vi "Clear Connections.vi"(8 "error in (no error)":errorcluster, 11 "RT Data Cluster in":T1={"Timekeeper hdl"="", "clkDisc session"=variant, "Compiled Data"={"SyncMod?"=FALSE, "SyncMod"="", "ConnectionSettings"={"Mode"=enum."Generate sample clock", "pxitrig"=FALSE, "pfi0"=FALSE, "pfi1"=FALSE, "pfi2"=FALSE, "External Pin"=enum."PFI0", "Routes"=[]}, "TimeKeeper"="", "ScanOffset(%)"=0.0, "StartDelay(s)"=0, "Time Ref Settings"={"Time Reference"=enum."GPS", "Priority 1"=0, "Priority 2"=0, "IRIG type"=enum."IRIGB AM", "Terminal"="", "PPSSetTime"=FALSE, "Start Time"=timestamp(0 s since 1904-01-01)}, "FIFO Locations"={"BoardTime"=[], "Status"=[]}}, "OutputsData"=[], "OutputsFIFO"=refnum, "Scan Period"=0, "Timekeeper type"=enum."6683", "SyncMod type"=enum."6683", "SyncMod hdl"="", "Custom Device Name"=""} {"Compiled Data"."Time Ref Settings"."Priority 2" min=0 max=255; "Compiled Data"."Time Ref Settings"."Priority 1" min=0 max=255}) -> (0 "error out":errorcluster, 3 "RT Data Cluster out":T1={"Timekeeper hdl"="", "clkDisc session"=variant, "Compiled Data"={"SyncMod?"=FALSE, "SyncMod"="", "ConnectionSettings"={"Mode"=enum."Generate sample clock", "pxitrig"=FALSE, "pfi0"=FALSE, "pfi1"=FALSE, "pfi2"=FALSE, "External Pin"=enum."PFI0", "Routes"=[]}, "TimeKeeper"="", "ScanOffset(%)"=0.0, "StartDelay(s)"=0, "Time Ref Settings"={"Time Reference"=enum."GPS", "Priority 1"=0, "Priority 2"=0, "IRIG type"=enum."IRIGB AM", "Terminal"="", "PPSSetTime"=FALSE, "Start Time"=timestamp(0 s since 1904-01-01)}, "FIFO Locations"={"BoardTime"=[], "Status"=[]}}, "OutputsData"=[], "OutputsFIFO"=refnum, "Scan Period"=0, "Timekeeper type"=enum."6683", "SyncMod type"=enum."6683", "SyncMod hdl"="", "Custom Device Name"=""} {"Compiled Data"."Time Ref Settings"."Priority 2" min=0 max=255; "Compiled Data"."Time Ref Settings"."Priority 1" min=0 max=255})   [LabVIEW 2020, in "NI Synchronization Engine.lvlib"]
uses:
  NI Synchronization Engine.lvlib
  Timekeeper Route Pin.ctl
  <instrlib>/niSync/niSync.llb/niSync Initialize (Default).vi
  niveristand-synchronization-custom-device-2024/Source/Engine/mdevClkDisc.llb/_clkDisc_session.ctl
  Shared/Route.ctl
  Shared/NI Synchronization Shared.lvlib
  Shared/Routes.ctl
  Shared/External Pin.ctl
  Shared/Mode.ctl
  Shared/Connection Settings.ctl
  Shared/IRIG Type.ctl
  Shared/Time Ref Settings.ctl
  Shared/Compiled Data.ctl
  RT Data Cluster.ctl
  Shared/Time Reference.ctl
  timekeeper type.ctl
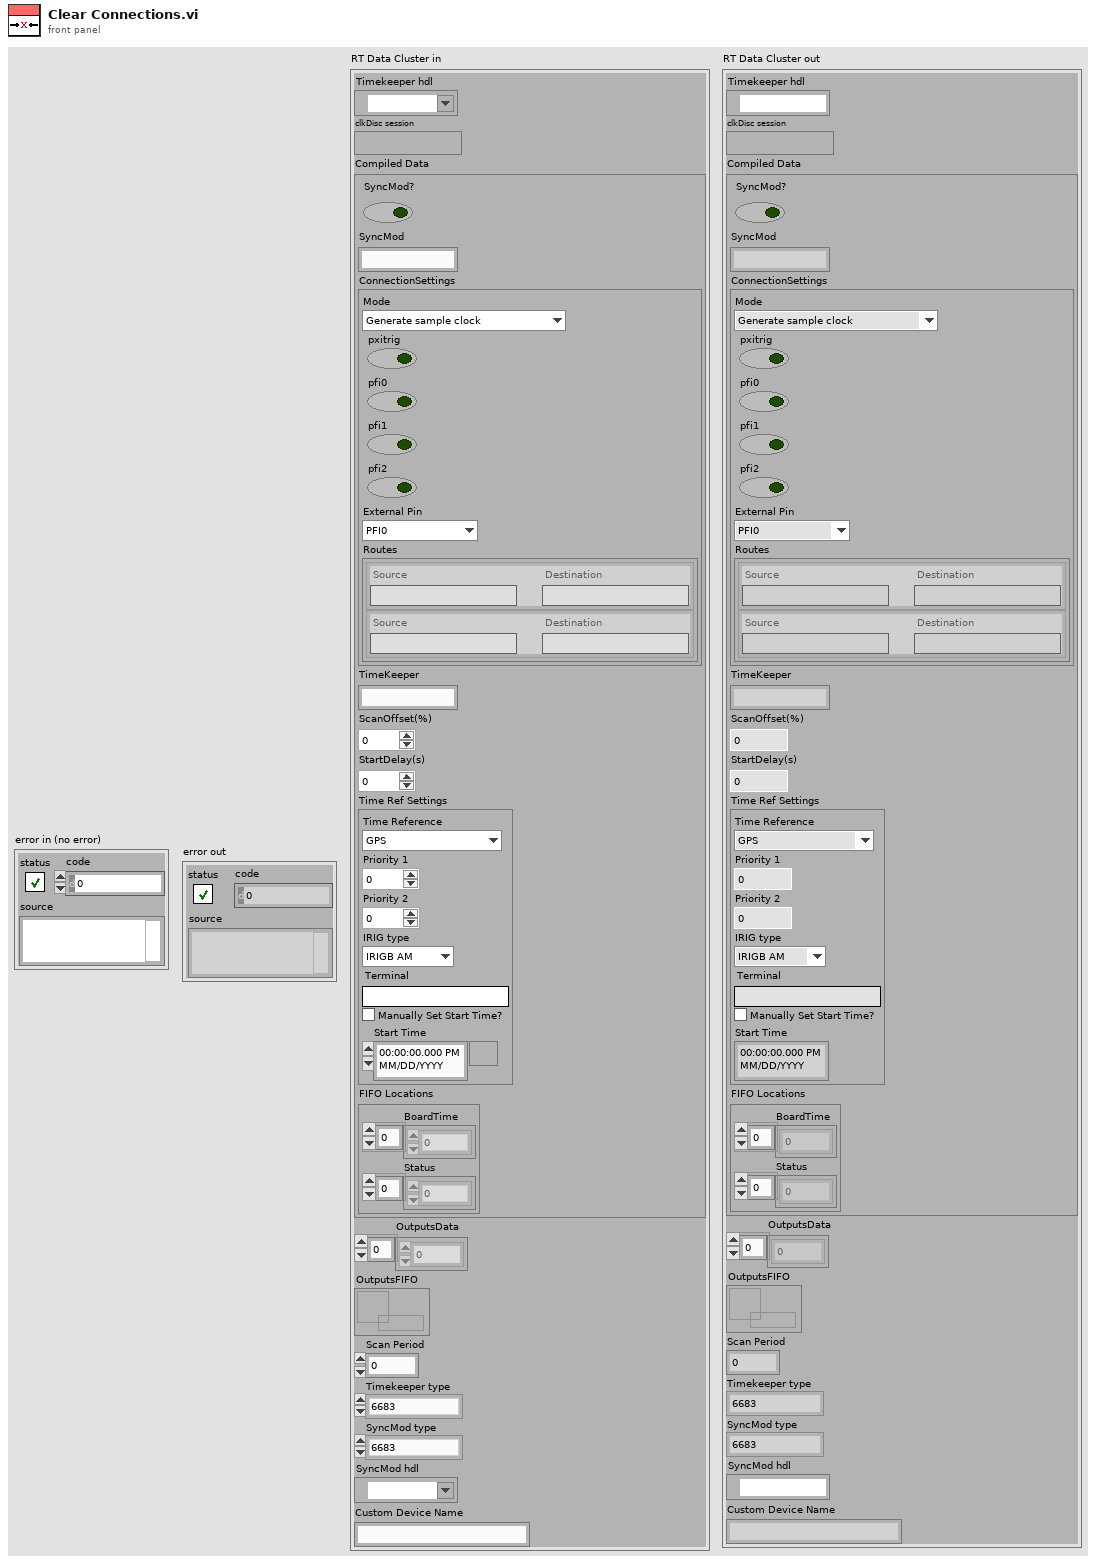
[diagram p1: front panel]
types:
  T1 = typedef "NI Synchronization Engine.lvlib/RT Data Cluster.ctl" = cluster{"Timekeeper hdl":refnum<k15>, "clkDisc session":T2, "Compiled Data":T3, "OutputsData":dbl[], "OutputsFIFO":refnum<k33>, "Scan Period":u32, "Timekeeper type":T12, "SyncMod type":T12, "SyncMod hdl":refnum<k15>, "Custom Device Name":string}
  T2 = typedef "_clkDisc_session.ctl" = variant
  T3 = typedef "NI Synchronization Shared.lvlib/Compiled Data.ctl" = cluster{"SyncMod?":bool, "SyncMod":string, "ConnectionSettings":T4, "TimeKeeper":string, "ScanOffset(%)":dbl, "StartDelay(s)":u16, "Time Ref Settings":T9, "FIFO Locations":cluster{"BoardTime":i32[], "Status":i32[]}}
  T4 = typedef "NI Synchronization Shared.lvlib/Connection Settings.ctl" = cluster{"Mode":T5, "pxitrig":bool, "pfi0":bool, "pfi1":bool, "pfi2":bool, "External Pin":T6, "Routes":T7}
  T5 = typedef "NI Synchronization Shared.lvlib/Mode.ctl" = enum16{"Generate sample clock", "Route sample clock out of chassis", "Route sample clock into chassis", "Custom routes"}
  T6 = typedef "NI Synchronization Shared.lvlib/External Pin.ctl" = enum16{"PFI0", "PFI1", "PFI2"}
  T7 = typedef "NI Synchronization Shared.lvlib/Routes.ctl" = T8[]
  T8 = typedef "NI Synchronization Shared.lvlib/Route.ctl" = cluster{"Source":string, "Destination":string}
  T9 = typedef "NI Synchronization Shared.lvlib/Time Ref Settings.ctl" = cluster{"Time Reference":T10, "Priority 1":i32, "Priority 2":i32, "IRIG type":T11, "Terminal":string, "PPSSetTime":bool, "Start Time":timestamp}
  T10 = typedef "NI Synchronization Shared.lvlib/Time Reference.ctl" = enum16{"GPS", "IRIG", "PPS", "1588 Ordinary Clock", "802.1AS", "PXI Chassis Clock", "Free Running (Internal)"}
  T11 = typedef "NI Synchronization Shared.lvlib/IRIG Type.ctl" = enum16{"IRIGB DC", "IRIGB AM"}
  T12 = typedef "NI Synchronization Engine.lvlib/timekeeper type.ctl" = enum16{"6683", "6683H", "6682", "6682H", "non-timekeeper", "timekeeper"}
  T13 = typedef "NI Synchronization Engine.lvlib/Timekeeper Route Pin.ctl" = enum16{"TTL0", "PFI0", "PFI1", "PFI2", "PXI_Clk10", "PXI_Clk10_In", "BoardClk", "ClkOut", "Oscillator"}
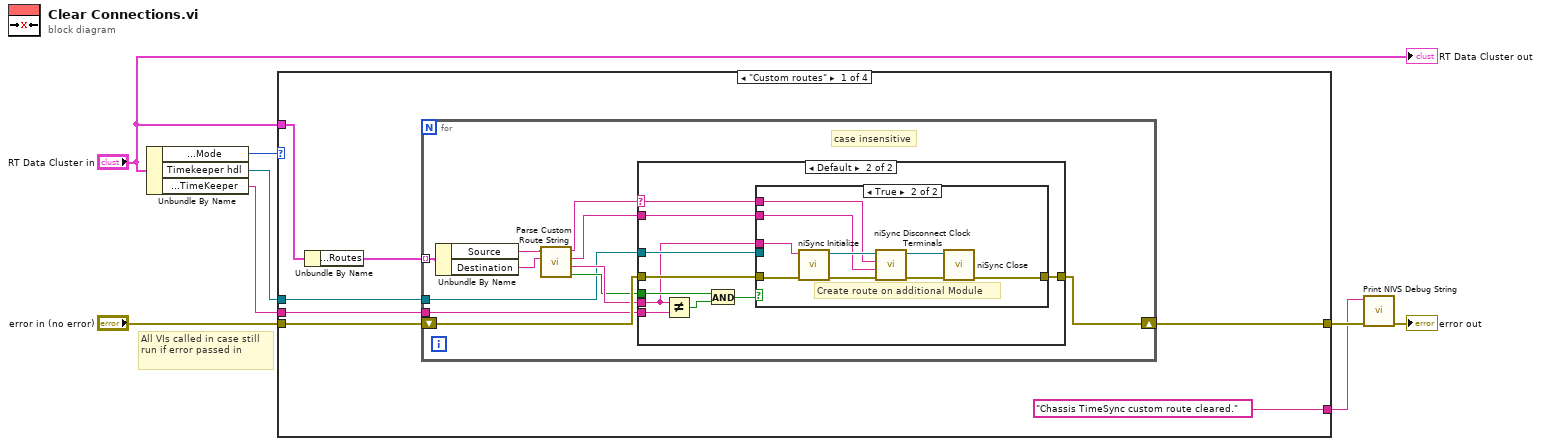
[diagram p0: block diagram]
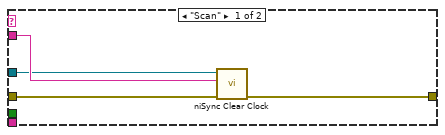
[diagram p2: hidden frame]
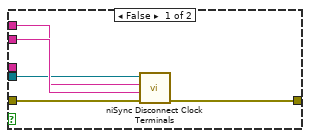
[diagram p3: hidden frame]
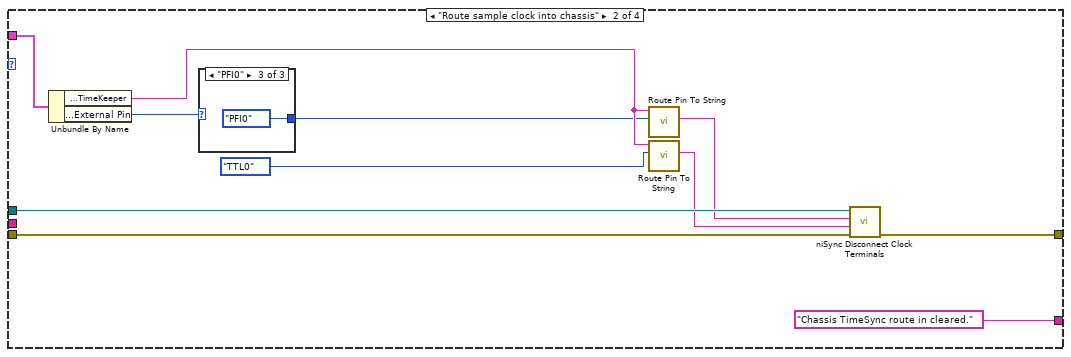
[diagram p4: hidden frame]
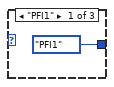
[diagram p5: hidden frame]
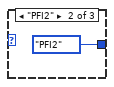
[diagram p6: hidden frame]
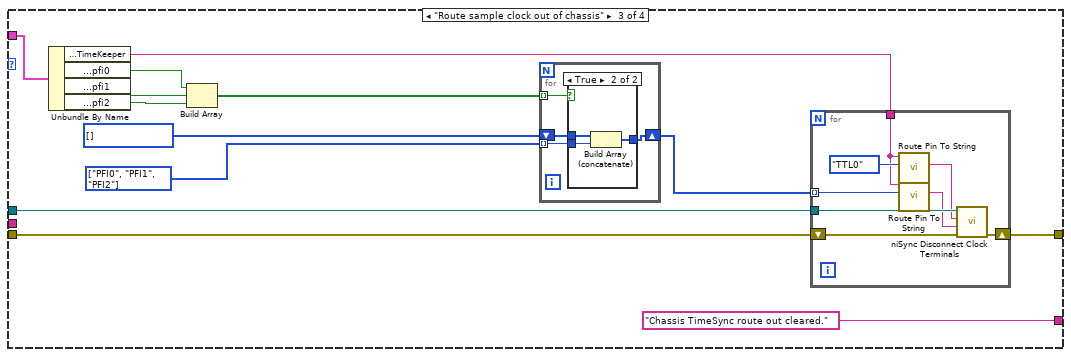
[diagram p7: hidden frame]
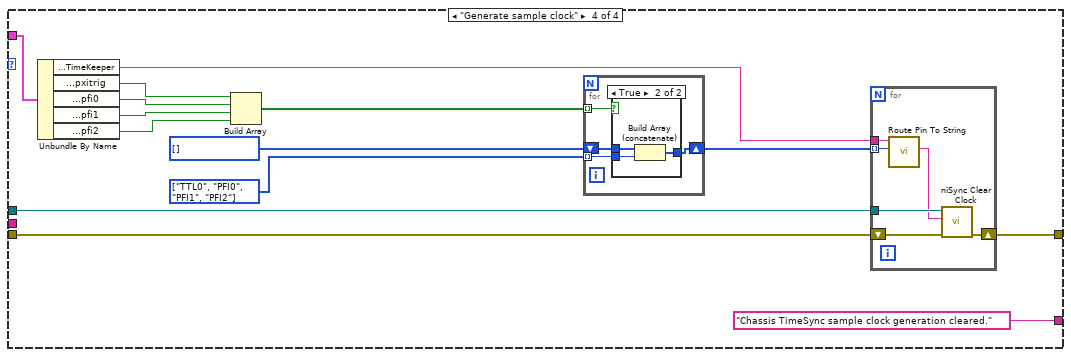
[diagram p9: hidden frame]
diagram:
  # "All VIs called in case still run if error passed in"
  n1 = Unbundle By Name("RT Data Cluster in") -> ("Compiled Data.ConnectionSettings.Mode"=w8:T5, "Timekeeper hdl"=w7:refnum<k15>, "Compiled Data.TimeKeeper"=w1:string)
  n2 = case shown="\"Custom routes\"" w8 {
    tunnel: w7 -> [w11 w59 w80 w111]
    tunnel: "RT Data Cluster in" -> [w15 w65 w81 w109]
    tunnel: [w12 w63 w70 w98] -> w5
    tunnel: ["Chassis TimeSync custom route cleared." "Chassis TimeSync route in cleared." "Chassis TimeSync route out cleared." "Chassis TimeSync sample clock generation cleared."] -> w4
    tunnel: "error in (no error)" -> [w10 w55 w69 w99]
    tunnel: w1 -> [w9 _ _ _]
    frame "Custom routes" {
      n3 = Unbundle By Name(w15) -> ("Compiled Data.ConnectionSettings.Routes"=w14:T7)
      n4 = for {
        tunnel: w14 -> [w26] mode=indexing
        tunnel: w11 -> [w17]
        shift-right: [w22] -> w12
        shift-left: w10 -> [w23]
        tunnel: w9 -> [w16]
        # "case insensitive"
        n5 = Unbundle By Name(w26) -> ("Source"=w25:string, "Destination"=w24:string)
        n6 = call "Parse Custom Route String.vi"("Destination In"=w24, "Source In"=w25) -> ("Module?"=w18:bool, "Module Out"=w19:string, "Destination Out"=w21:string, "Source Out"=w20:string)  [unwired: 6 in]
        n7 = case shown="Default" w20 {
          selector: w20 -> [_ w36]
          tunnel: w23 -> [w29 w40]
          tunnel: w21 -> [w28 w39]
          tunnel: [w30 w38] -> w22
          tunnel: w17 -> [w27 w37]
          tunnel: w18 -> [_ w34]
          tunnel: w19 -> [_ w32]
          tunnel: w16 -> [_ w31]
          frame "Scan" {
            n8 = call <instrlib>:"niSync Clear Clock.vi"("error in (no error)"=w29, "terminal"=w28, "instrument handle"=w27) -> ("error out"=w30:errorcluster)  [unwired: 6 in, 1 out]
          }
          frame Default {
            n9 = Not Equal?(x=w32, y=w31) -> (x != y?=w33:bool)
            n10 = And(x=w34, y=w33) -> (x .and. y?=w35:bool)
            n11 = case shown="True" w35 {
              tunnel: w40 -> [w45 w52]
              tunnel: w39 -> [w44 w48]
              tunnel: [w43 w46] -> w38
              tunnel: w37 -> [w42 _]
              tunnel: w36 -> [w41 w49]
              tunnel: w32 -> [_ w51]
              frame False {
                n12 = call <instrlib>:"niSync Disconnect Clock Terminals.vi"("error in (no error)"=w45, "destination terminal"=w44, "source terminal"=w41, "instrument handle"=w42) -> ("error out"=w43:errorcluster)  [unwired: 6 in, 1 out]
              }
              frame True {
                # "Create route on additional Module"
                n13 = call-poly <instrlib>:"niSync Initialize.vi"("error in (no error)"=w52, "resource name"=w51) -> ("error out"=w54:errorcluster, "instrument handle out"=w50:refnum<k15>)  [unwired: 8 in]
                n14 = call <instrlib>:"niSync Disconnect Clock Terminals.vi"("error in (no error)"=w54, "destination terminal"=w48, "source terminal"=w49, "instrument handle"=w50) -> ("error out"=w53:errorcluster, "instrument handle out"=w47:refnum<k15>)  [unwired: 6 in]
                n15 = call <instrlib>:"niSync Close.vi"("error in (no error)"=w53, "instrument handle"=w47) -> ("error out"=w46:errorcluster)  [unwired: 9 in]
              }
            }
          }
        }
      }
    }
    frame "Route sample clock into chassis" {
      n16 = Unbundle By Name(w65) -> ("Compiled Data.TimeKeeper"=w62:string, "Compiled Data.ConnectionSettings.External Pin"=w64:T6)
      n17 = case shown="\"PFI0\"" w64 {
        tunnel: [Timekeeper_Route_Pin."PFI1" ("Pin") Timekeeper_Route_Pin."PFI2" ("Pin") Timekeeper_Route_Pin."PFI0" ("Pin")] -> w60
        frame "PFI1" {
        }
        frame "PFI2" {
        }
        frame "PFI0" {
        }
      }
      n18 = call "Route Pin To String.vi"("Pin"=w60, "Module"=w62) -> ("String"=w58:string)  [unwired: 9 in]
      n19 = call "Route Pin To String.vi"("Pin"=Timekeeper_Route_Pin."TTL0", "Module"=w62) -> ("String"=w57:string)  [unwired: 9 in]
      n20 = call <instrlib>:"niSync Disconnect Clock Terminals.vi"("error in (no error)"=w55, "destination terminal"=w57, "source terminal"=w58, "instrument handle"=w59) -> ("error out"=w63:errorcluster)  [unwired: 6 in, 1 out]
    }
    frame "Route sample clock out of chassis" {
      w73 = T13[] [enum."PFI0", enum."PFI1", enum."PFI2"] items=["TTL0", "PFI0", "PFI1", "PFI2", "PXI_Clk10", "PXI_Clk10_In", "BoardClk", "ClkOut", "Oscillator"]
      w74 = T13[] [] items=["TTL0", "PFI0", "PFI1", "PFI2", "PXI_Clk10", "PXI_Clk10_In", "BoardClk", "ClkOut", "Oscillator"]
      n21 = Unbundle By Name(w81) -> ("Compiled Data.TimeKeeper"=w79:string, "Compiled Data.ConnectionSettings.pfi0"=w78:bool, "Compiled Data.ConnectionSettings.pfi1"=w77:bool, "Compiled Data.ConnectionSettings.pfi2"=w76:bool)
      n22 = Build Array(w78, w77, w76) -> (w75:bool[])
      n23 = for {
        tunnel: w75 -> [w85] mode=indexing
        shift-right: [w82] -> w72
        shift-left: w74 -> [w84]
        tunnel: w73 -> [w83] mode=indexing
        n24 = case shown="True" w85 {
          tunnel: w84 -> [w86 w89]
          tunnel: w83 -> [_ w88]
          tunnel: [w86 w87] -> w82
          frame False {
          }
          frame True {
            n25 = Build Array (concatenate)(w89, w88) -> (w87:T13[])
          }
        }
      }
      n26 = for {
        tunnel: w80 -> [w97]
        tunnel: w79 -> [w94]
        tunnel: w72 -> [w92] mode=indexing
        shift-right: [w91] -> w70
        shift-left: w69 -> [w90]
        n27 = call "Route Pin To String.vi"("Pin"=Timekeeper_Route_Pin."TTL0", "Module"=w94) -> ("String"=w96:string)  [unwired: 9 in]
        n28 = call "Route Pin To String.vi"("Pin"=w92, "Module"=w94) -> ("String"=w93:string)  [unwired: 9 in]
        n29 = call <instrlib>:"niSync Disconnect Clock Terminals.vi"("error in (no error)"=w90, "destination terminal"=w93, "source terminal"=w96, "instrument handle"=w97) -> ("error out"=w91:errorcluster)  [unwired: 6 in, 1 out]
      }
    }
    frame "Generate sample clock" {
      w106 = T13[] [enum."TTL0", enum."PFI0", enum."PFI1", enum."PFI2"] items=["TTL0", "PFI0", "PFI1", "PFI2", "PXI_Clk10", "PXI_Clk10_In", "BoardClk", "ClkOut", "Oscillator"]
      w107 = T13[] [] items=["TTL0", "PFI0", "PFI1", "PFI2", "PXI_Clk10", "PXI_Clk10_In", "BoardClk", "ClkOut", "Oscillator"]
      n30 = Unbundle By Name(w109) -> ("Compiled Data.TimeKeeper"=w104:string, "Compiled Data.ConnectionSettings.pxitrig"=w103:bool, "Compiled Data.ConnectionSettings.pfi0"=w102:bool, "Compiled Data.ConnectionSettings.pfi1"=w101:bool, "Compiled Data.ConnectionSettings.pfi2"=w100:bool)
      n31 = Build Array(w103, w102, w101, w100) -> (w108:bool[])
      n32 = for {
        tunnel: w108 -> [w115] mode=indexing
        shift-right: [w112] -> w105
        shift-left: w107 -> [w114]
        tunnel: w106 -> [w113] mode=indexing
        n33 = case shown="True" w115 {
          tunnel: w114 -> [w116 w119]
          tunnel: w113 -> [_ w118]
          tunnel: [w116 w117] -> w112
          frame False {
          }
          frame True {
            n34 = Build Array (concatenate)(w119, w118) -> (w117:T13[])
          }
        }
      }
      n35 = for {
        tunnel: w111 -> [w125]
        tunnel: w105 -> [w124] mode=indexing
        tunnel: w104 -> [w122]
        shift-right: [w121] -> w98
        shift-left: w99 -> [w120]
        n36 = call "Route Pin To String.vi"("Pin"=w124, "Module"=w122) -> ("String"=w123:string)  [unwired: 9 in]
        n37 = call <instrlib>:"niSync Clear Clock.vi"("error in (no error)"=w120, "terminal"=w123, "instrument handle"=w125) -> ("error out"=w121:errorcluster)  [unwired: 6 in, 1 out]
      }
    }
  }
  n38 = call "Print NIVS Debug String.vi"("error in (no error)"=w5, "Debug String"=w4) -> ("error out"=→"error out":errorcluster)  [unwired: 8 in]
  "RT Data Cluster out" <- "RT Data Cluster in"
